vi "test_ao-1ch1pt.vi"() -> ()   [LabVIEW 2019]
panel:
  out "vo":i32
  in  "y":i32=6
  out "error out":errorcluster caption="에러 출력"
  in  "dt":u32=400
  in  "정지":bool
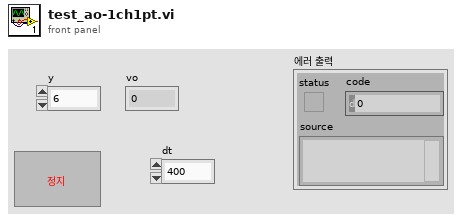
[diagram p1: front panel]
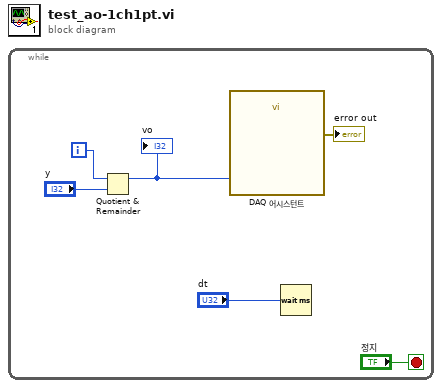
[diagram p0: block diagram]
diagram:
  n1 = while {
    i -> [w4]
    stop <- "정지" stop-if-true
    n2 = Quotient & Remainder(x=w4, y="y") -> (x-y*floor(x/y)=w2:i32)  [unwired: 1 out]
    "vo" <- w2
    n3 = call "DAQ 어시스턴트"("data"=w2) -> ("error out"=→"error out":errorcluster)  [unwired: 17 in, 1 out]
    n4 = Wait (ms)(milliseconds to wait="dt") -> ()  [unwired: 1 out]
  }
